vi "rs3 wait for frames4.vi"(8 "error in (no error)":errorcluster, 10 "timeout":u32=1000, 11 "Queue in":u64) -> (0 "error out":errorcluster, 1 "frame":u64, 2 "error out":u64, 3 "queue out":u64)   [LabVIEW 2017, in "libRealSense3.lvlib"]
doc: "Block until new frames are available. Returns the next FRAME handle when available."
uses:
  libRealSense3.lvlib
panel:
  # "RS3 Wait for Frame"
  # "(C) Intel Corp. 2017,  AGJ"
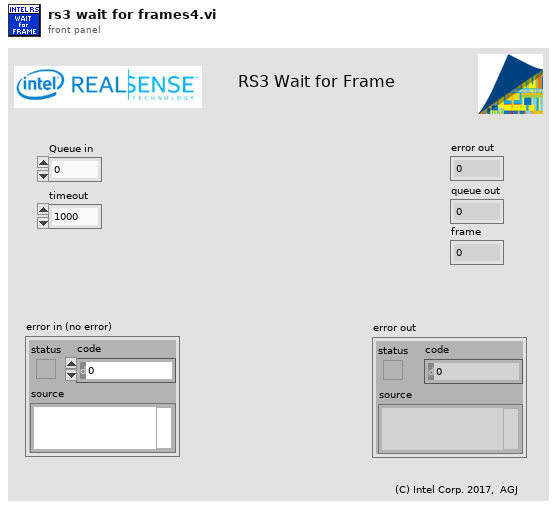
[diagram p1: front panel]
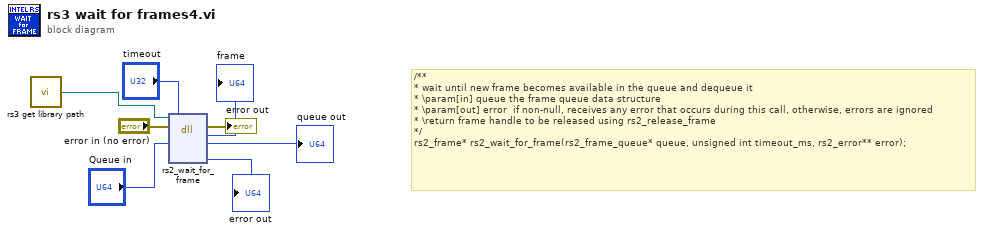
[diagram p0: block diagram]
diagram:
  # "/**\n* wait until new frame becomes available in the queue and dequeue it\n* \\param[in] queue the frame queue data structure\n* \\param[out] error  if non-null, receives any error that occurs during this call, otherwise, errors are ignored\n* \\return frame handle to be released using rs2_release_frame\n*/\nrs2_frame* rs2_wait_for_frame(rs2_frame_queue* queue, unsigned int timeout_ms, rs2_error** error);"
  n1 = call "rs3 get library path.vi"() -> ("Realsense 2 Library Path"=w1:path)
  n2 = dll-call lib="C:/Users/agrunnet/Documents/libRealSense6/realsense2.dll" fn="rs2_wait_for_frame"(path in=w1, error in="error in (no error)", "queue in"="Queue in", "timeout"="timeout") -> (error out=→"error out":errorcluster, "frame"=→"frame":u64, "queue in"=→"queue out":u64, "error"=→"error out":u64)  [unwired: 3 in, 1 out]
